vi "GetUserFramePosition.vi"(8 "group":i32, 9 "userFrame":i32, 10 "Snpx":refnum<k24>, 11 "error in":errorcluster) -> (0 "UserTool":i16, 1 "Cartesian position":T1, 2 "JointsPosition":dbl[](array[numeric]), 3 "error out":errorcluster)   [LabVIEW 2022 SP3, in "UnderAutomation.Fanuc.lvlib"]
uses:
  UnderAutomation.Fanuc.lvlib
  C:/Users/fg/Documents/Fanuc.vi/LabVIEW_2024/UnderAutomation.Fanuc/lib/UnderAutomation.Fanuc.dll
  LabVIEW_2024/UnderAutomation.Fanuc/lib/UnderAutomation.Fanuc.dll
panel:
  out "UserFrame":i16
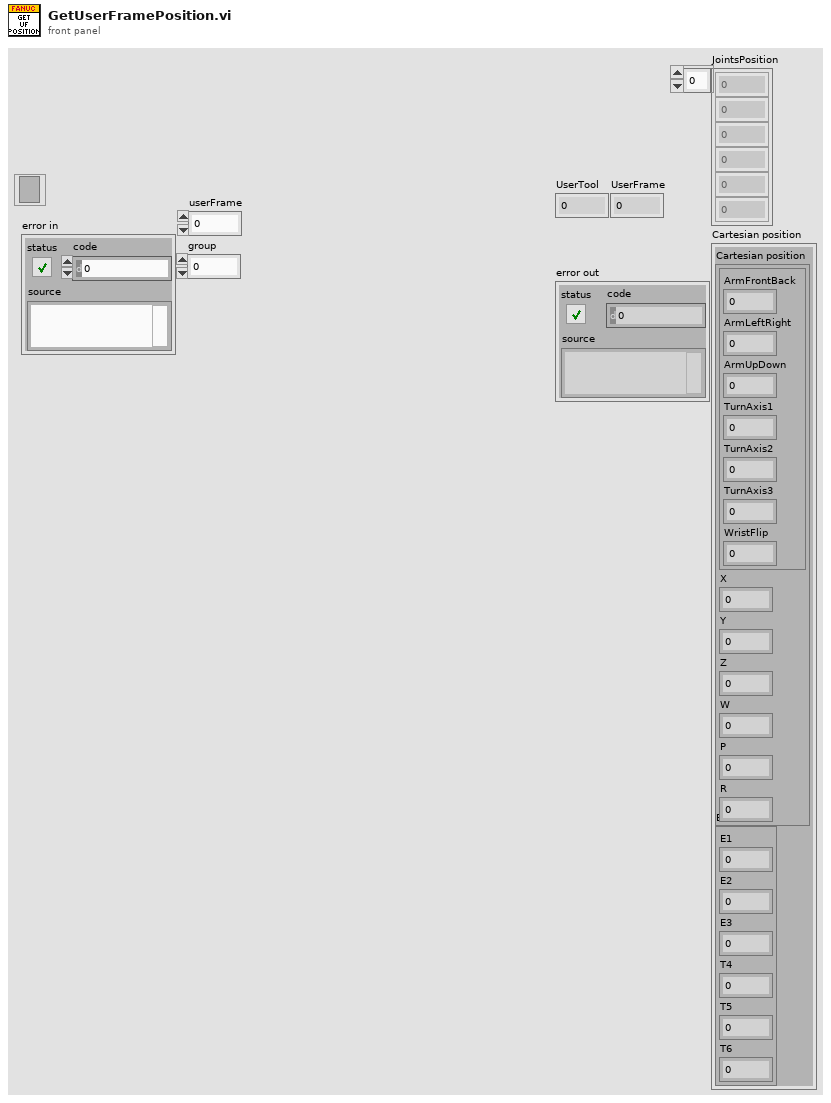
[diagram p1: front panel]
types:
  T1 = cluster{"Cartesian position":cluster{cluster{"ArmFrontBack":i32, "ArmLeftRight":i32, "ArmUpDown":i32, "TurnAxis1":i32, "TurnAxis2":i32, "TurnAxis3":i32, "WristFlip":i32}, "X":dbl, "Y":dbl, "Z":dbl, "W":dbl, "P":dbl, "R":dbl}, "Extension":cluster{"E1":dbl, "E2":dbl, "E3":dbl, "T4":i16, "T5":i16, "T6":i16}}
  T2 = cluster{"Configuration":cluster{"ArmFrontBack":i32, "ArmLeftRight":i32, "ArmUpDown":i32, "TurnAxis1":i32, "TurnAxis2":i32, "TurnAxis3":i32, "WristFlip":i32}, "X":dbl, "Y":dbl, "Z":dbl, "W":dbl, "P":dbl, "R":dbl}
  T3 = cluster{"E1":dbl, "E2":dbl, "E3":dbl, "T4":i16, "T5":i16, "T6":i16}
  T4 = cluster{"Cartesian position":cluster{"Configuration":cluster{"ArmFrontBack":i32, "ArmLeftRight":i32, "ArmUpDown":i32, "TurnAxis1":i32, "TurnAxis2":i32, "TurnAxis3":i32, "WristFlip":i32}, "X":dbl, "Y":dbl, "Z":dbl, "W":dbl, "P":dbl, "R":dbl}, cluster{"E1":dbl, "E2":dbl, "E3":dbl, "T4":i16, "T5":i16, "T6":i16}}
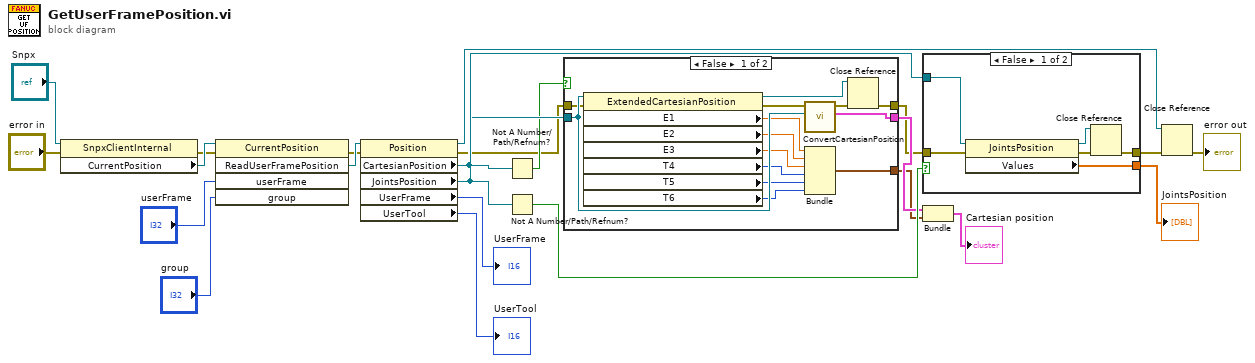
[diagram p0: block diagram]
diagram:
  n1 = property class="SnpxClientInternal"(reference="Snpx", error in="error in") -> (error out=w20:errorcluster, "CurrentPosition"=w21:refnum<k24>)  [unwired: 1 out]
  n2 = invoke class="CurrentPosition" method="ReadUserFramePosition"(reference=w21, error in=w20, "userFrame"="userFrame", "group"="group") -> (error out=w4:errorcluster, "ReadUserFramePosition"=w19:refnum<k24>)  [unwired: 1 in, 3 out]
  n3 = property class="Position"(reference=w19, error in=w4) -> (reference out=w18:refnum<k24>, error out=w7:errorcluster, "CartesianPosition"=w12:refnum<k24>, "JointsPosition"=w14:refnum<k24>, "UserFrame"=→"UserFrame":i16, "UserTool"=→"UserTool":i16)
  n4 = Not A Number/Path/Refnum?(number/path/refnum=w12) -> (NaN/Path/Refnum?=w11:bool)
  n5 = Not A Number/Path/Refnum?(number/path/refnum=w14) -> (NaN/Path/Refnum?=w15:bool)
  n6 = case shown="False" w11 {
    tunnel: w12 -> [w36 _]
    tunnel: [w37 _] -> w10
    tunnel: [w29 _] -> w9
    tunnel: w7 -> [w28 w38]
    tunnel: [w26 w38] -> w6
    frame False {
      n7 = property class="ExtendedCartesianPosition"(reference=w36, error in=w28) -> (reference out=w27:refnum<k24>, error out=w25:errorcluster, "E1"=w35:dbl, "E2"=w34:dbl, "E3"=w33:dbl, "T4"=w32:i16, "T5"=w31:i16, "T6"=w30:i16)
      n8 = call "ConvertCartesianPosition.vi"("Cartesian position"=w36, "error in (no error)"=w25) -> ("Cartesian position"=w37:T2, "error out"=w24:errorcluster)  [unwired: 8 in]
      n9 = Bundle("E1"=w35, "E2"=w34, "E3"=w33, "T4"=w32, "T5"=w31, "T6"=w30) -> (w29:T3)  [unwired: 1 in]
      n10 = Close Reference(reference=w27, error in (no error)=w24) -> (error out=w26:errorcluster)
    }
    frame True {
    }
  }
  n11 = case shown="False" w15 {
    tunnel: w14 -> [w44 _]
    tunnel: [w43 _] -> w13
    tunnel: w6 -> [w40 w45]
    tunnel: [w39 w45] -> w5
    frame False {
      n12 = property class="JointsPosition"(reference=w44, error in=w40) -> (reference out=w41:refnum<k24>, error out=w42:errorcluster, "Values"=w43:dbl[])
      n13 = Close Reference(reference=w41, error in (no error)=w42) -> (error out=w39:errorcluster)
    }
    frame True {
    }
  }
  "JointsPosition" <- w13
  n14 = Bundle("Cartesian position"=w10, w9) -> (→"Cartesian position":T4)  [unwired: 1 in]
  n15 = Close Reference(reference=w18, error in (no error)=w5) -> (error out=→"error out":errorcluster)
